vi "release queue.vi"(8 "error in (no error)":errorcluster caption="에러 입력(에러 없음)", 11 "GUI Log Class 입력":refnum<class "GUI Log Class.lvclass">) -> (0 "error out":errorcluster caption="에러 출력", 3 "GUI Log Class 출력":refnum<class "GUI Log Class.lvclass">)   [LabVIEW 2020, in "GUI Log Class.lvclass"]
uses:
  GUI Log Class.lvclass
  GUI Log Class.lvclass/GUI Log Class.ctl
  Accessors/Read appender queue.vi
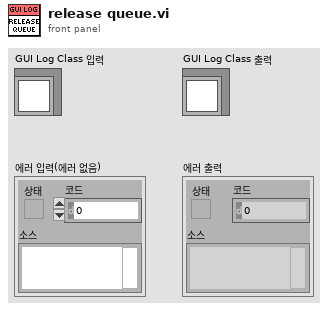
[diagram p1: front panel]
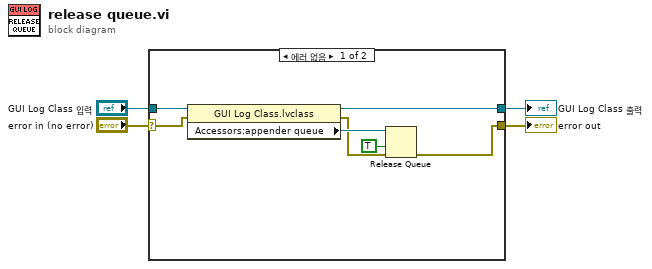
[diagram p0: block diagram]
diagram:
  n1 = case shown="에러 없음" "error in (no error)" {
    selector: "error in (no error)" -> [w9 w13]
    tunnel: [w6 w13] -> w3
    tunnel: [w10 w12] -> w1
    tunnel: "GUI Log Class 입력" -> [w11 w12]
    frame No Error {
      n2 = property class="GUI Log Class.lvclass"(reference=w11, error in=w9) -> (reference out=w10:refnum<class "GUI Log Class.lvclass">, error out=w7:errorcluster, "Accessors:appender queue"=w8:refnum<queue>)
      n3 = Release Queue(queue=w8, force destroy? (F)=TRUE ("강제 삭제? (거짓)"), error in (no error)=w7) -> (error out=w6:errorcluster)  [unwired: 2 out]
    }
    frame Error {
    }
  }
  "error out" <- w3
  "GUI Log Class 출력" <- w1
